vi "subBluetoothConnect.vi"(8 "error in (no error)":errorcluster) -> (0 "error out":errorcluster, 2 "Log":string[](array[string]), 3 "Number of Wiimotes Connected":i32)   [LabVIEW 2011]
uses:
  C:/Users/whitemrj/Dropbox/RHRT LabVIEW/Robot Prodcution Code/Sprint 4/Working Code 2/Remote/Wiimote/Wiimote/InTheHand.Net.Personal.dll
  InTheHand.Net.Personal.dll
panel:
  in  "System.Timespan":refnum<k24>
  in  "Listbox":i32(listbox)
  in  "Bluetooth Security":refnum<k24>
  in  "Bluetooth Service":refnum<k24>
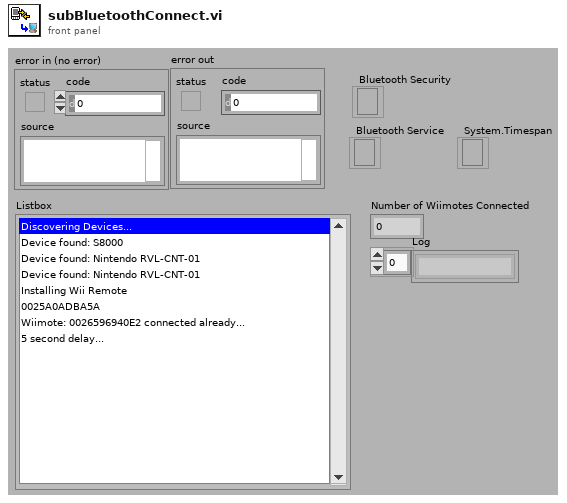
[diagram p1: front panel]
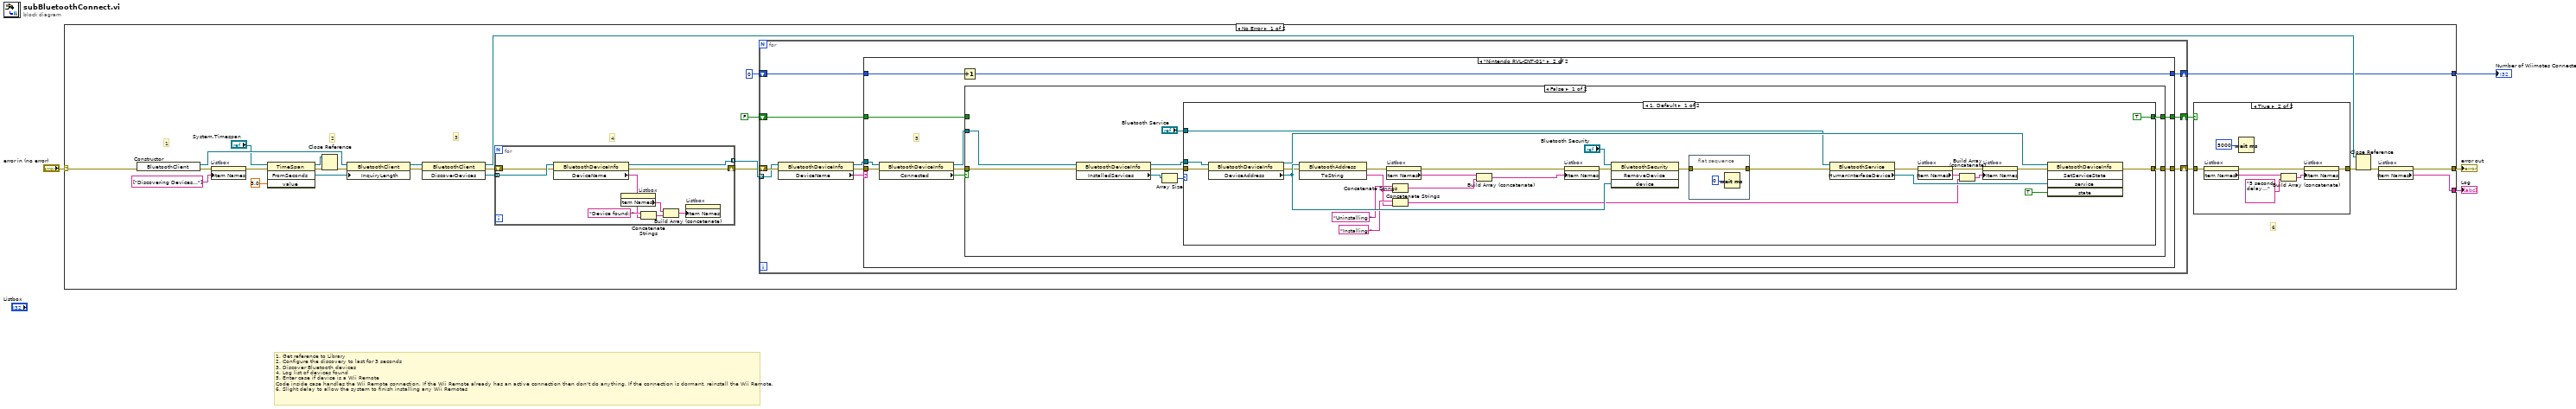
[diagram p0: block diagram]
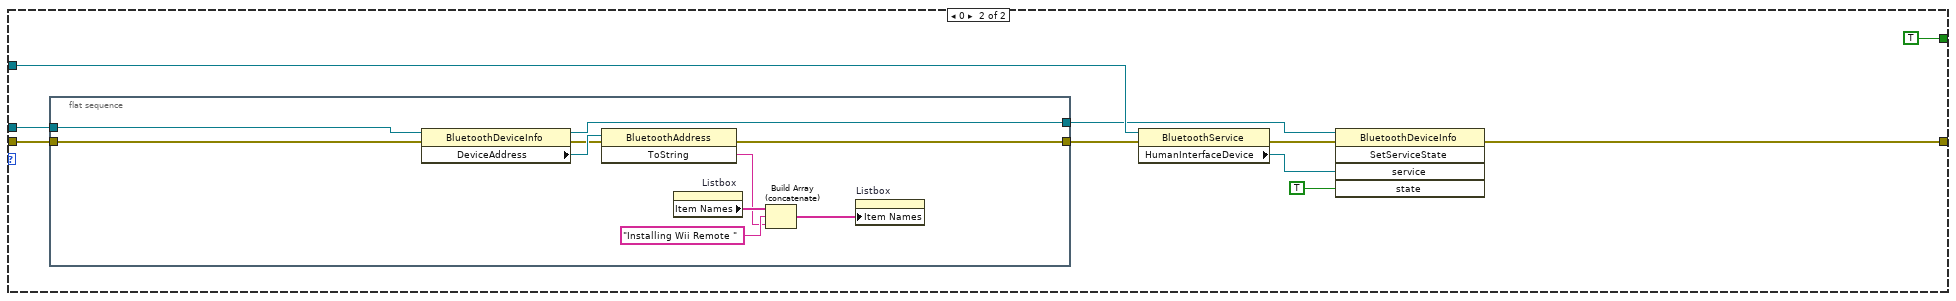
[diagram p4: hidden frame]
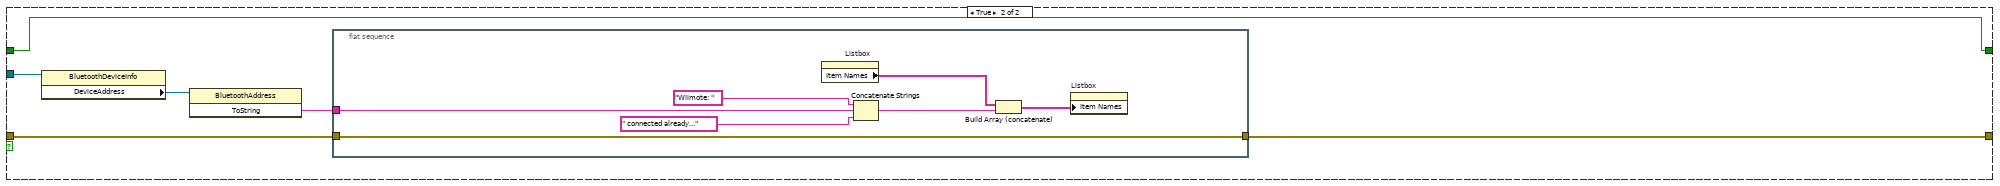
[diagram p5: hidden frame]
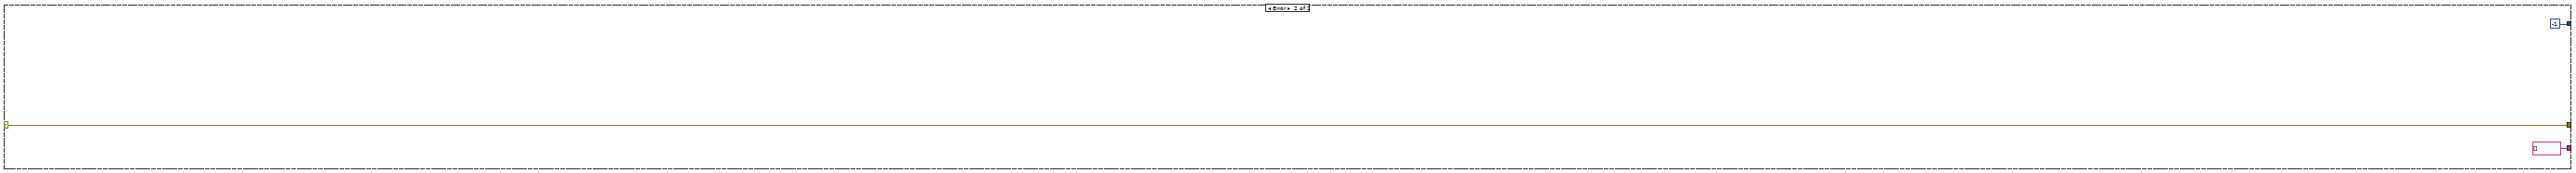
[diagram p6: hidden frame]
diagram:
  # "1. Get reference to Library\n2. Configure the discovery to last for 3 seconds\n3. Discover Bluetooth devices\n4. Log list of devices found\n5. Enter case if device is a Wii Remote\nCode inside case handles the Wii Remote connection. If the Wii Remote already has an active connection then don't do anything. If the connection is dormant, reinstall the Wii Remote.\n6. Slight delay to allow the system to finish installing any Wii Remotes"
  n1 = case shown="No Error" "error in (no error)" {
    selector: "error in (no error)" -> [w16 w146]
    tunnel: [w18 w146] -> w1
    tunnel: [w17 string[] [] ("Item Names")] -> w4
    tunnel: [w15 -1] -> w2
    frame No Error {
      # "6"
      # "4"
      # "3"
      # "2"
      # "1"
      n2 = constructor class="BluetoothClient"(error in=w16) -> (reference out=w14:refnum<k24>, error out=w21:errorcluster)  [unwired: 2 in, 1 out]
      n3 = property on="Listbox" class="LstBox (strict)"(error in=w21, "Item Names"=string[] ["Discovering Devices..."]) -> (error out=w5:errorcluster)  [unwired: 1 in, 1 out]
      n4 = invoke class="TimeSpan" method="FromSeconds"(reference="System.Timespan", error in=w5, "value"=3.0) -> (reference out=w9:refnum<k24>, error out=w8:errorcluster, "FromSeconds"=w10:refnum<k24>)  [unwired: 1 in, 1 out]
      n5 = Close Reference(reference=w9, error in (no error)=w8) -> (error out=w7:errorcluster)
      n6 = property class="BluetoothClient"(reference=w14, error in=w7, "InquiryLength"=w10) -> (reference out=w13:refnum<k24>, error out=w6:errorcluster)
      n7 = invoke class="BluetoothClient" method="DiscoverDevices"(reference=w13, error in=w6) -> (reference out=w31:refnum<k24>, error out=w22:errorcluster, "DiscoverDevices"=w26:refnum<k24>[])  [unwired: 1 in]
      n8 = for {
        tunnel: w26 -> [w40] mode=indexing
        tunnel: [w39] -> w25 mode=indexing
        shift-right: [w38] -> w24
        shift-left: w22 -> [w37]
        n9 = property class="BluetoothDeviceInfo"(reference=w40, error in=w37) -> (reference out=w39:refnum<k24>, error out=w38:errorcluster, "DeviceName"=w32:string)
        n10 = property on="Listbox" class="LstBox (strict)"() -> ("Item Names"=w36:string[])  [unwired: 2 in, 2 out]
        n11 = Concatenate Strings("Device found: ", w32) -> (w34:string)
        n12 = Build Array (concatenate)(w36, w34) -> (w35:string[])
        n13 = property on="Listbox" class="LstBox (strict)"("Item Names"=w35) -> ()  [unwired: 2 in, 2 out]
      }
      n14 = for {
        shift-right: [w55] -> w27
        shift-left: w24 -> [w56]
        tunnel: w25 -> [w53] mode=indexing
        shift-right: [w52] -> w29
        shift-left: FALSE -> [w51]
        shift-right: [w49] -> w15
        shift-left: 0 -> [w50]
        n15 = property class="BluetoothDeviceInfo"(reference=w53, error in=w56) -> (reference out=w57:refnum<k24>, error out=w54:errorcluster, "DeviceName"=w58:string)
        n16 = case shown="\"Nintendo RVL-CNT-01\"" w58 {
          tunnel: w57 -> [_ w71]
          tunnel: [w61 w68] -> w55
          tunnel: w54 -> [w61 w67]
          tunnel: [w60 w65] -> w52
          tunnel: w51 -> [w60 w64]
          tunnel: w50 -> [w59 w63]
          tunnel: [w59 w62] -> w49
          frame "", Default {
          }
          frame "Nintendo RVL-CNT-01" {
            # "5"
            n17 = property class="BluetoothDeviceInfo"(reference=w71, error in=w67) -> (reference out=w69:refnum<k24>, error out=w66:errorcluster, "Connected"=w70:bool)
            n18 = Increment(x=w63) -> (x+1=w62:i32)
            n19 = case shown="False" w70 {
              tunnel: w69 -> [w80 w134]
              tunnel: [w75 w135] -> w68
              tunnel: w66 -> [w74 w136]
              tunnel: [w72 w131] -> w65
              tunnel: w64 -> [_ w131]
              frame False {
                n20 = property class="BluetoothDeviceInfo"(reference=w80, error in=w74) -> (reference out=w77:refnum<k24>, error out=w73:errorcluster, "InstalledServices"=w79:refnum<k24>[])
                n21 = Array Size(array=w79) -> (size(s)=w78:i32)
                n22 = case shown="1, Default" w78 {
                  tunnel: w77 -> [w107 w112]
                  tunnel: "Bluetooth Service" -> [w103 w118]
                  tunnel: [w81 w116] -> w75
                  tunnel: w73 -> [w101 w114]
                  tunnel: [TRUE ("state") TRUE ("state")] -> w72
                  frame 1, Default {
                    n23 = property class="BluetoothDeviceInfo"(reference=w107, error in=w101) -> (reference out=w104:refnum<k24>, error out=w99:errorcluster, "DeviceAddress"=w100:refnum<k24>)
                    n24 = invoke class="BluetoothAddress" method="ToString"(reference=w100, error in=w99) -> (error out=w86:errorcluster, "ToString"=w88:string)  [unwired: 1 in, 1 out]
                    n25 = property on="Listbox" class="LstBox (strict)"(error in=w86) -> (error out=w93:errorcluster, "Item Names"=w95:string[])  [unwired: 1 in, 1 out]
                    n26 = Concatenate Strings("Uninstalling ", w88) -> (w90:string)
                    n27 = Concatenate Strings("Installing ", w88) -> (w87:string)
                    n28 = Build Array (concatenate)(w95, w90) -> (w94:string[])
                    n29 = property on="Listbox" class="LstBox (strict)"(error in=w93, "Item Names"=w94) -> (error out=w85:errorcluster)  [unwired: 1 in, 1 out]
                    n30 = invoke class="BluetoothSecurity" method="RemoveDevice"(reference="Bluetooth Security", error in=w85, "device"=w100) -> (error out=w84:errorcluster)  [unwired: 1 in, 3 out]
                    n31 = flat-sequence {
                      tunnel: w84 -> [w109]
                      tunnel: [w109] -> w92
                      frame #0 {
                        n32 = Wait (ms)(milliseconds to wait=u32 0) -> ()  [unwired: 1 out]
                      }
                    }
                    n33 = property class="BluetoothService"(reference=w103, error in=w92) -> (error out=w83:errorcluster, "HumanInterfaceDevice"=w105:refnum<k24>)  [unwired: 1 out]
                    n34 = property on="Listbox" class="LstBox (strict)"(error in=w83) -> (error out=w96:errorcluster, "Item Names"=w97:string[])  [unwired: 1 in, 1 out]
                    n35 = Build Array (concatenate)(w97, w87) -> (w98:string[])
                    n36 = property on="Listbox" class="LstBox (strict)"(error in=w96, "Item Names"=w98) -> (error out=w82:errorcluster)  [unwired: 1 in, 1 out]
                    n37 = invoke class="BluetoothDeviceInfo" method="SetServiceState"(reference=w104, error in=w82, "service"=w105, "state"=TRUE) -> (error out=w81:errorcluster)  [unwired: 1 in, 4 out]
                  }
                  frame 0 {
                    n38 = flat-sequence {
                      tunnel: [w121] -> w115
                      tunnel: w114 -> [w122]
                      tunnel: w112 -> [w126]
                      tunnel: [w125] -> w111
                      frame #0 {
                        n39 = property class="BluetoothDeviceInfo"(reference=w126, error in=w122) -> (reference out=w125:refnum<k24>, error out=w123:errorcluster, "DeviceAddress"=w127:refnum<k24>)
                        n40 = invoke class="BluetoothAddress" method="ToString"(reference=w127, error in=w123) -> (error out=w121:errorcluster, "ToString"=w124:string)  [unwired: 1 in, 1 out]
                        n41 = property on="Listbox" class="LstBox (strict)"() -> ("Item Names"=w129:string[])  [unwired: 2 in, 2 out]
                        n42 = Build Array (concatenate)(w129, "Installing Wii Remote " ("Status"), w124) -> (w128:string[])
                        n43 = property on="Listbox" class="LstBox (strict)"("Item Names"=w128) -> ()  [unwired: 2 in, 2 out]
                      }
                    }
                    n44 = property class="BluetoothService"(reference=w118, error in=w115) -> (error out=w117:errorcluster, "HumanInterfaceDevice"=w119:refnum<k24>)  [unwired: 1 out]
                    n45 = invoke class="BluetoothDeviceInfo" method="SetServiceState"(reference=w111, error in=w117, "service"=w119, "state"=TRUE) -> (error out=w116:errorcluster)  [unwired: 1 in, 4 out]
                  }
                }
              }
              frame True {
                n46 = property class="BluetoothDeviceInfo"(reference=w134) -> ("DeviceAddress"=w133:refnum<k24>)  [unwired: 1 in, 2 out]
                n47 = invoke class="BluetoothAddress" method="ToString"(reference=w133) -> ("ToString"=w132:string)  [unwired: 2 in, 2 out]
                n48 = flat-sequence {
                  tunnel: [w143] -> w135
                  tunnel: w136 -> [w143]
                  tunnel: w132 -> [w142]
                  frame #0 {
                    n49 = property on="Listbox" class="LstBox (strict)"() -> ("Item Names"=w138:string[])  [unwired: 2 in, 2 out]
                    n50 = Concatenate Strings("Wiimote: " ("string"), w142, " connected already..." ("string")) -> (w139:string)
                    n51 = Build Array (concatenate)(w138, w139) -> (w137:string[])
                    n52 = property on="Listbox" class="LstBox (strict)"("Item Names"=w137) -> ()  [unwired: 2 in, 2 out]
                  }
                }
              }
            }
          }
        }
      }
      n53 = case shown="True" w29 {
        tunnel: [w41 w44] -> w28
        tunnel: w27 -> [w41 w43]
        frame False {
        }
        frame True {
          n54 = property on="Listbox" class="LstBox (strict)"(error in=w43) -> (error out=w42:errorcluster, "Item Names"=w47:string[])  [unwired: 1 in, 1 out]
          n55 = Wait (ms)(milliseconds to wait=u32 5000) -> ()  [unwired: 1 out]
          n56 = Build Array (concatenate)(w47, "5 second delay..." ("Status")) -> (w45:string[])
          n57 = property on="Listbox" class="LstBox (strict)"(error in=w42, "Item Names"=w45) -> (error out=w44:errorcluster)  [unwired: 1 in, 1 out]
        }
      }
      n58 = Close Reference(reference=w31, error in (no error)=w28) -> (error out=w19:errorcluster)
      n59 = property on="Listbox" class="LstBox (strict)"(error in=w19) -> (error out=w18:errorcluster, "Item Names"=w17:string[])  [unwired: 1 in, 1 out]
    }
    frame Error {
    }
  }
  "error out" <- w1
  "Log" <- w4
  "Number of Wiimotes Connected" <- w2
